vi "FIR Filtering and Response.vi"() -> ()   [LabVIEW 2020]
doc: "Filters an input signal using the Finite Impulse Response (FIR) filter design technique. You can specify the type of the filter, such as low pass or band pass; filter topology, such as Equi-ripple or Windowed FIR; and filter specifications, such as filter order or cutoff frequency. You can feed a single channel or multiple channels to the Digital FIR Filter VI used in this example."
uses:
  <vilib>/measure/macond.llb/FIR Filter by N Specs for N Chan.vi
  <vilib>/measure/macond.llb/FIR Filter for N Chan.vi
  <vilib>/measure/macond.llb/FIR Filter for 1 Chan.vi
  <vilib>/measure/NI_MABase.lvlib
  <vilib>/measure/NI_MAPro.lvlib
panel:
  in  "Configuration":T1(tab)
  in  "signal parameters":T2={"signal type"=enum."Sine Wave", "frequency"=101.0} {"frequency" format="%#.6g"}
  in  "sampling info":cluster{"Fs":dbl, "#s":dbl}={"Fs"=1000.0, "#s"=100.0} {"#s" step=100.0 format="%#.6g"; "Fs" step=1000.0 format="%0.2p"}
  in  "FIR filter specifications":T3={"Topology"=enum."Equi-ripple FIR", "Type"=enum."Lowpass", "#Taps"=50, "Lower PB"=100.0, "Upper PB"=0.0, "Lower SB"=200.0, "Upper SB"=0.0} {"Upper SB" format="%#.6g"; "Lower SB" format="%#.6g"; "Upper PB" format="%#.6g"; "Lower PB" format="%#.6g"}
  in  "reset signal":bool
  in  "reset filter":bool
  in  "N-waveforms 1-filter":T4(array[cluster])=[{"reset signal"=FALSE, "signal parameters"={"signal type"=enum."Sine Wave", "frequency"=101.0}, "sampling info"={"Fs"=1000.0, "#s"=100.0}}, {"reset signal"=FALSE, "signal parameters"={"signal type"=enum."Sine Wave", "frequency"=101.0}, "sampling info"={"Fs"=1000.0, "#s"=100.0}}] {"sampling info"."#s" step=100.0 format="%#.6g"; "sampling info"."Fs" step=1000.0 format="%0.2p"; "signal parameters"."frequency" format="%#.6g"}
  in  "FIR filter specifications":T3={"Topology"=enum."Equi-ripple FIR", "Type"=enum."Lowpass", "#Taps"=50, "Lower PB"=100.0, "Upper PB"=0.0, "Lower SB"=200.0, "Upper SB"=0.0} {"Upper SB" format="%#.6g"; "Lower SB" format="%#.6g"; "Upper PB" format="%#.6g"; "Lower PB" format="%#.6g"}
  in  "reset filter":bool
  in  "reset filter":bool
  in  "N-waveforms N-filters":T5(array[cluster])=[{"signal parameters"={"signal type"=enum."Sine Wave", "frequency"=101.0}, "sampling info"={"Fs"=1000.0, "#s"=100.0}, "FIR filter specifications"={"Topology"=enum."Equi-ripple FIR", "Type"=enum."Lowpass", "#Taps"=50, "Lower PB"=100.0, "Upper PB"=0.0, "Lower SB"=200.0, "Upper SB"=0.0}, "reset signal"=FALSE}, {"signal parameters"={"signal type"=enum."Sine Wave", "frequency"=101.0}, "sampling info"={"Fs"=1000.0, "#s"=100.0}, "FIR filter specifications"={"Topology"=enum."Equi-ripple FIR", "Type"=enum."Lowpass", "#Taps"=50, "Lower PB"=100.0, "Upper PB"=0.0, "Lower SB"=200.0, "Upper SB"=0.0}, "reset signal"=FALSE}] {"FIR filter specifications"."Upper SB" format="%#.6g"; "FIR filter specifications"."Lower SB" format="%#.6g"; "FIR filter specifications"."Upper PB" format="%#.6g"; "FIR filter specifications"."Lower PB" format="%#.6g"; "sampling info"."#s" step=100.0 format="%#.6g"; "sampling info"."Fs" step=1000.0 format="%#.6g"; "signal parameters"."frequency" format="%#.6g"}
  in  "Graphs":T6(tab)
  out "Waveform Graph":waveform(dbl)[](graph)
  out "Magnitude response":cluster{"f0":dbl, "df":dbl, "Mag H(w)":dbl[]}(graph)={"f0"=0.0, "df"=0.9765625, "Mag H(w)"=[]}
  out "Phase response":cluster{"f0":dbl, "df":dbl, "Phase H(w)":dbl[]}(graph)={"f0"=0.0, "df"=0.9765625, "Phase H(w)"=[]}
  in  "Stop":bool
  # "Overview: This example demonstrates the different polymorphic instances of the Digital FIR Filter VI.\nRequirements: LabVIEW Full Development System\nInstructions:\n1. Run the VI.\n2. Select different tabs.\n3. Interact with the filter specifications and signal parameters.\n4. Click Stop to stop the VI."
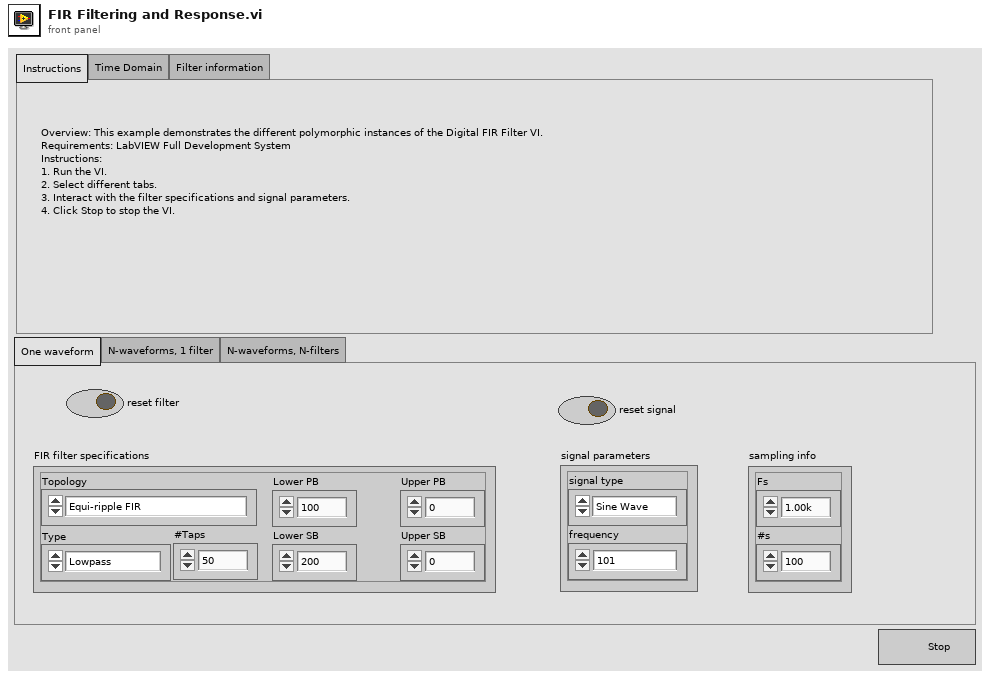
[diagram p1: front panel]
types:
  T1 = enum32{"One waveform", "N-waveforms, 1 filter", "N-waveforms, N-filters"}
  T2 = cluster{"signal type":enum16{"Sine Wave", "Triangle Wave", "Square Wave", "Sawtooth Wave"}, "frequency":dbl}
  T3 = cluster{"Topology":enum16{"Off", "FIR by Specification", "Equi-ripple FIR", "Windowed FIR"}, "Type":enum16{"Lowpass", "Highpass", "Bandpass", "Bandstop"}, "#Taps":i32, "Lower PB":dbl, "Upper PB":dbl, "Lower SB":dbl, "Upper SB":dbl}
  T4 = cluster{"reset signal":bool, "signal parameters":cluster{"signal type":enum16{"Sine Wave", "Triangle Wave", "Square Wave", "Sawtooth Wave"}, "frequency":dbl}, "sampling info":cluster{"Fs":dbl, "#s":dbl}}[]
  T5 = cluster{"signal parameters":cluster{"signal type":enum16{"Sine Wave", "Triangle Wave", "Square Wave", "Sawtooth Wave"}, "frequency":dbl}, "sampling info":cluster{"Fs":dbl, "#s":dbl}, "FIR filter specifications":cluster{"Topology":enum16{"Off", "FIR by Specification", "Equi-ripple FIR", "Windowed FIR"}, "Type":enum16{"Lowpass", "Highpass", "Bandpass", "Bandstop"}, "#Taps":i32, "Lower PB":dbl, "Upper PB":dbl, "Lower SB":dbl, "Upper SB":dbl}, "reset signal":bool}[]
  T6 = enum32{"Instructions", "Time Domain", "Filter information"}
  T7 = cluster{"magnitude H(w)":cluster{"f0":dbl, "df":dbl, "Mag H(w)":dbl[]}, "phase H(w)":cluster{"f0":dbl, "df":dbl, "Phase H(w)":dbl[]}, "order":i32}[]
  T8 = cluster{"magnitude H(w)":cluster{"f0":dbl, "df":dbl, "Mag H(w)":dbl[]}, "phase H(w)":cluster{"f0":dbl, "df":dbl, "Phase H(w)":dbl[]}, "order":i32}
  T9 = enum16{"Sine Wave", "Triangle Wave", "Square Wave", "Sawtooth Wave"}
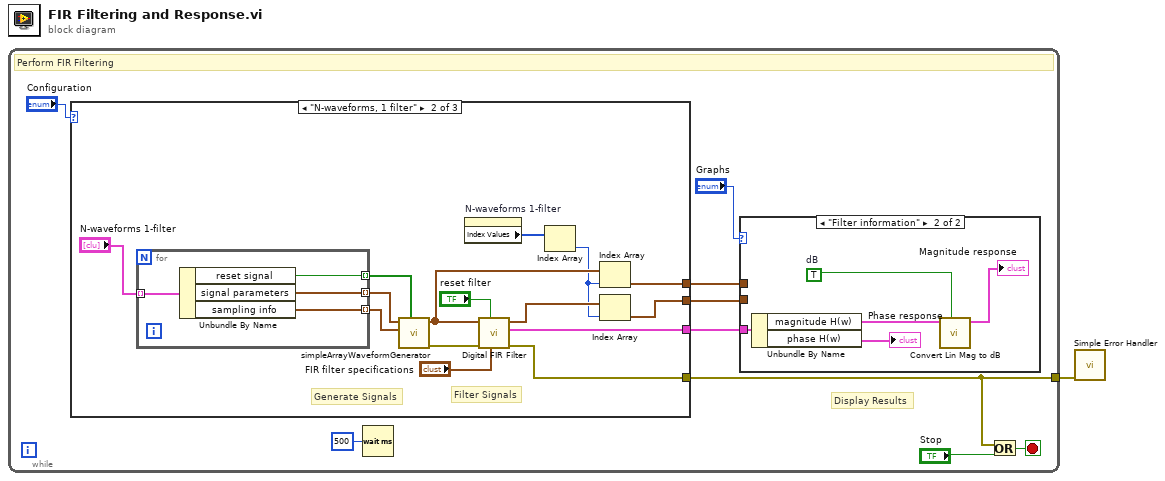
[diagram p0: block diagram]
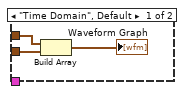
[diagram p2: hidden frame]
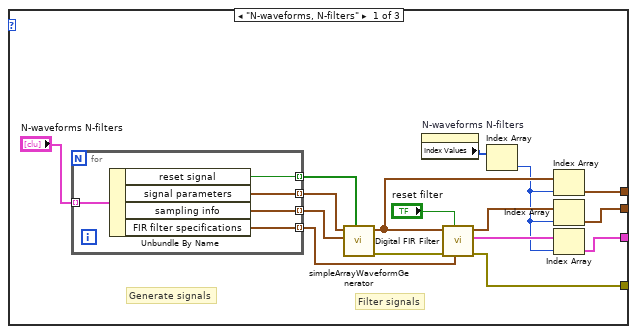
[diagram p3: hidden frame]
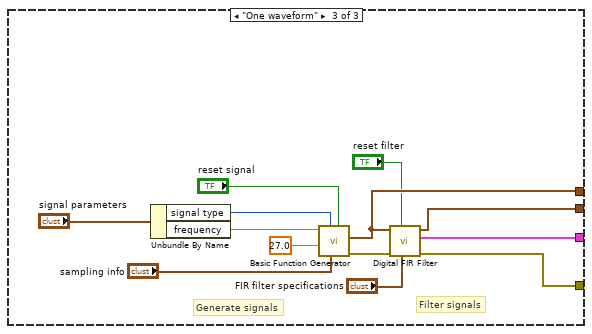
[diagram p4: hidden frame]
diagram:
  n1 = while {
    tunnel: [w2] -> w1
    stop <- w9 stop-if-true
    # "Display Results"
    # "Perform FIR Filtering"
    n2 = case shown="\"N-waveforms, 1 filter\"" "Configuration" {
      tunnel: [w34 w54 w71] -> w2
      tunnel: [w33 w53 w68] -> w6
      tunnel: [w32 w52 w67] -> w5
      tunnel: [w29 w50 w69] -> w7
      frame "N-waveforms, N-filters" {
        # "Filter signals"
        # "Generate signals"
        n3 = for {
          tunnel: "N-waveforms N-filters" -> [w39] mode=indexing
          tunnel: [w38] -> w25 mode=indexing
          tunnel: [w37] -> w24 mode=indexing
          tunnel: [w36] -> w23 mode=indexing
          tunnel: [w35] -> w19 mode=indexing
          n4 = Unbundle By Name(w39) -> ("reset signal"=w38:bool, "signal parameters"=w37:T2, "sampling info"=w36:cluster{"Fs":dbl, "#s":dbl}, "FIR filter specifications"=w35:T3)
        }
        n5 = call "simpleArrayWaveformGenerator.vi"("reset signal"=w25, "sampling info"=w23, "signal parameters"=w24) -> ("error out"=w27:errorcluster, "signal(s) in"=w28:waveform(dbl)[])  [unwired: 7 in]
        n6 = property on="N-waveforms N-filters" class="Arr (strict)"() -> ("Index Values"=w22:u32[])  [unwired: 2 in, 2 out]
        n7 = call-poly <vilib>:"Digital FIR Filter.vi"("FIR filter specifications"=w19, "reset filters"="reset filter", "error in (no error)"=w27, "signal(s) in"=w28) -> ("error out"=w34:errorcluster, "filter information"=w30:T7, "signal(s) out"=w31:waveform(dbl)[])  [unwired: 5 in]
        n8 = Index Array(array=w22) -> (element=w21:u32)  [unwired: 1 in]
        n9 = Index Array(array=w28, index=w21) -> (element=w33:waveform(dbl))
        n10 = Index Array(array=w31, index=w21) -> (element=w32:waveform(dbl))
        n11 = Index Array(array=w30, index=w21) -> (element=w29:T8)
      }
      frame "N-waveforms, 1 filter" {
        # "Filter Signals"
        # "Generate Signals"
        n12 = for {
          tunnel: "N-waveforms 1-filter" -> [w58] mode=indexing
          tunnel: [w57] -> w46 mode=indexing
          tunnel: [w56] -> w45 mode=indexing
          tunnel: [w55] -> w44 mode=indexing
          n13 = Unbundle By Name(w58) -> ("reset signal"=w57:bool, "signal parameters"=w56:T2, "sampling info"=w55:cluster{"Fs":dbl, "#s":dbl})
        }
        n14 = call "simpleArrayWaveformGenerator.vi"("reset signal"=w46, "sampling info"=w44, "signal parameters"=w45) -> ("error out"=w49:errorcluster, "signal(s) in"=w48:waveform(dbl)[])  [unwired: 7 in]
        n15 = property on="N-waveforms 1-filter" class="Arr (strict)"() -> ("Index Values"=w43:u32[])  [unwired: 2 in, 2 out]
        n16 = call-poly <vilib>:"Digital FIR Filter.vi"("FIR filter specifications"="FIR filter specifications", "reset filters"="reset filter", "error in (no error)"=w49, "signal(s) in"=w48) -> ("error out"=w54:errorcluster, "filter information"=w50:T8, "signal(s) out"=w51:waveform(dbl)[])  [unwired: 5 in]
        n17 = Index Array(array=w43) -> (element=w42:u32)  [unwired: 1 in]
        n18 = Index Array(array=w48, index=w42) -> (element=w53:waveform(dbl))
        n19 = Index Array(array=w51, index=w42) -> (element=w52:waveform(dbl))
      }
      frame "One waveform" {
        # "Filter signals"
        # "Generate signals"
        n20 = Unbundle By Name("signal parameters") -> ("signal type"=w66:T9, "frequency"=w65:dbl)
        n21 = call <vilib>:"Basic Function Generator.vi"("reset signal"="reset signal", "sampling info"="sampling info", "signal type"=w66, "phase"=27.0, "frequency"=w65) -> ("error out"=w70:errorcluster, "signal out"=w68:waveform(dbl))  [unwired: 4 in, 1 out]
        n22 = call-poly <vilib>:"Digital FIR Filter.vi"("FIR filter specifications"="FIR filter specifications", "reset filter"="reset filter", "error in (no error)"=w70, "signal in"=w68) -> ("error out"=w71:errorcluster, "filter information"=w69:T8, "signal out"=w67:waveform(dbl))  [unwired: 5 in]
      }
    }
    n23 = Wait (ms)(milliseconds to wait=u32 500) -> ()  [unwired: 1 out]
    n24 = case shown="\"Filter information\"" "Graphs" {
      tunnel: w7 -> [_ w18]
      tunnel: w6 -> [w13 _]
      tunnel: w5 -> [w12 _]
      frame "Time Domain", Default {
        n25 = Build Array(w13, w12) -> (→"Waveform Graph":waveform(dbl)[])
      }
      frame "Filter information" {
        w14 = TRUE  # dB
        n26 = Unbundle By Name(w18) -> ("magnitude H(w)"=w17:cluster{"f0":dbl, "df":dbl, "Mag H(w)":dbl[]}, "phase H(w)"=→"Phase response":cluster{"f0":dbl, "df":dbl, "Phase H(w)":dbl[]})
        n27 = call "Convert Lin Mag to dB.vi"("convert to dB"=w14, "magnitude H(w)"=w17) -> ("magnitude H(w) in dB"=→"Magnitude response":cluster{"f0":dbl, "df":dbl, "Mag H(w)":dbl[]})  [unwired: 9 in]
      }
    }
    n28 = Or(x=w2, y="Stop") -> (x .or. y?=w9:bool)
  }
  n29 = call <vilib>:"Simple Error Handler.vi"("error in (no error)"=w1) -> ()  [unwired: 4 in, 5 out]
